vi "send_book_status.vi"(8 "error in (no error)":errorcluster, 10 "book status":T1, 11 "librarian in":refnum<class "librarian.lvclass">) -> (0 "error out":errorcluster, 3 "librarian out":refnum<class "librarian.lvclass">)   [LabVIEW 2020, in "librarian.lvclass"]
uses:
  librarian.lvclass
  typedefs/lib_map_value--cluster.ctl
  typedefs/book_state--enum.ctl
  librarian.lvclass/librarian.ctl
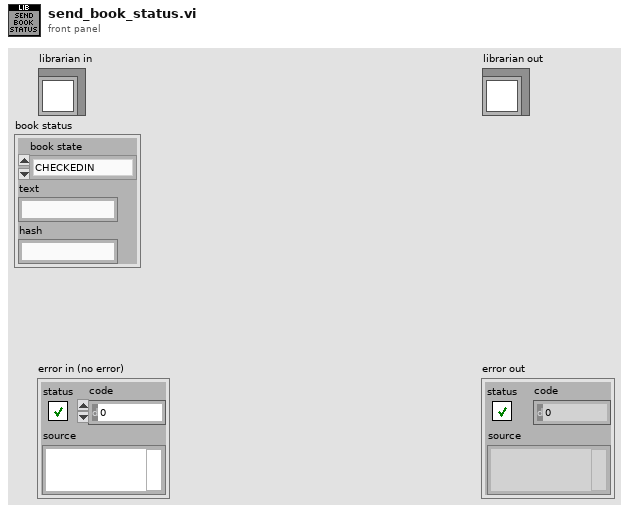
[diagram p1: front panel]
types:
  T1 = typedef "librarian.lvclass/lib_map_value--cluster.ctl" = cluster{"book state":T2, "text":string, "hash":string}
  T2 = typedef "librarian.lvclass/book_state--enum.ctl" = enum16{"CHECKEDIN", "CHECKEDOUT", "DAMAGED"}
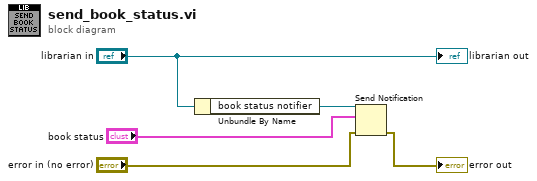
[diagram p0: block diagram]
diagram:
  n1 = Unbundle By Name("librarian in") -> ("book status notifier"=w4:refnum<notifier>)
  n2 = Send Notification(notification="book status", notifier=w4, error in (no error)="error in (no error)") -> (error out=→"error out":errorcluster)  [unwired: 1 out]
  "librarian out" <- "librarian in"
